vi "Retest.vi"(0 "Image In":T1, 1 "Image Dst":T1, 7 "error in":errorcluster) -> (20 "Image Out":T1, 21 "Objects (pixel) (Object Tracking 1)":T2(array[cluster]), 22 "Objects (real-world) (Object Tracking 1)":T2(array[cluster]), 27 "error out":errorcluster)   [LabVIEW 2016]
doc: "Creates, edits, and runs vision algorithms using NI Vision Assistant.\n\nWhen you place this Express VI on the block diagram, NI Vision Assistant launches. Create an algorithm using the Vision Assistant processing functions. After you create an algorithm, you can select the controls and indicators that you want to be able to programmatically set in LabVIEW. Double-click the Vision Assistant Express VI to edit the algorithm."
uses:
  <vilib>/vision/Image Controls.llb/IMAQ Image.ctl
  <vilib>/vision/Tracking.llb/IMAQ Object Tracking SessionType.ctl
  <vilib>/vision/Vision Assistant Utils.llb/IVA Object Tracking - Init Function.ctl
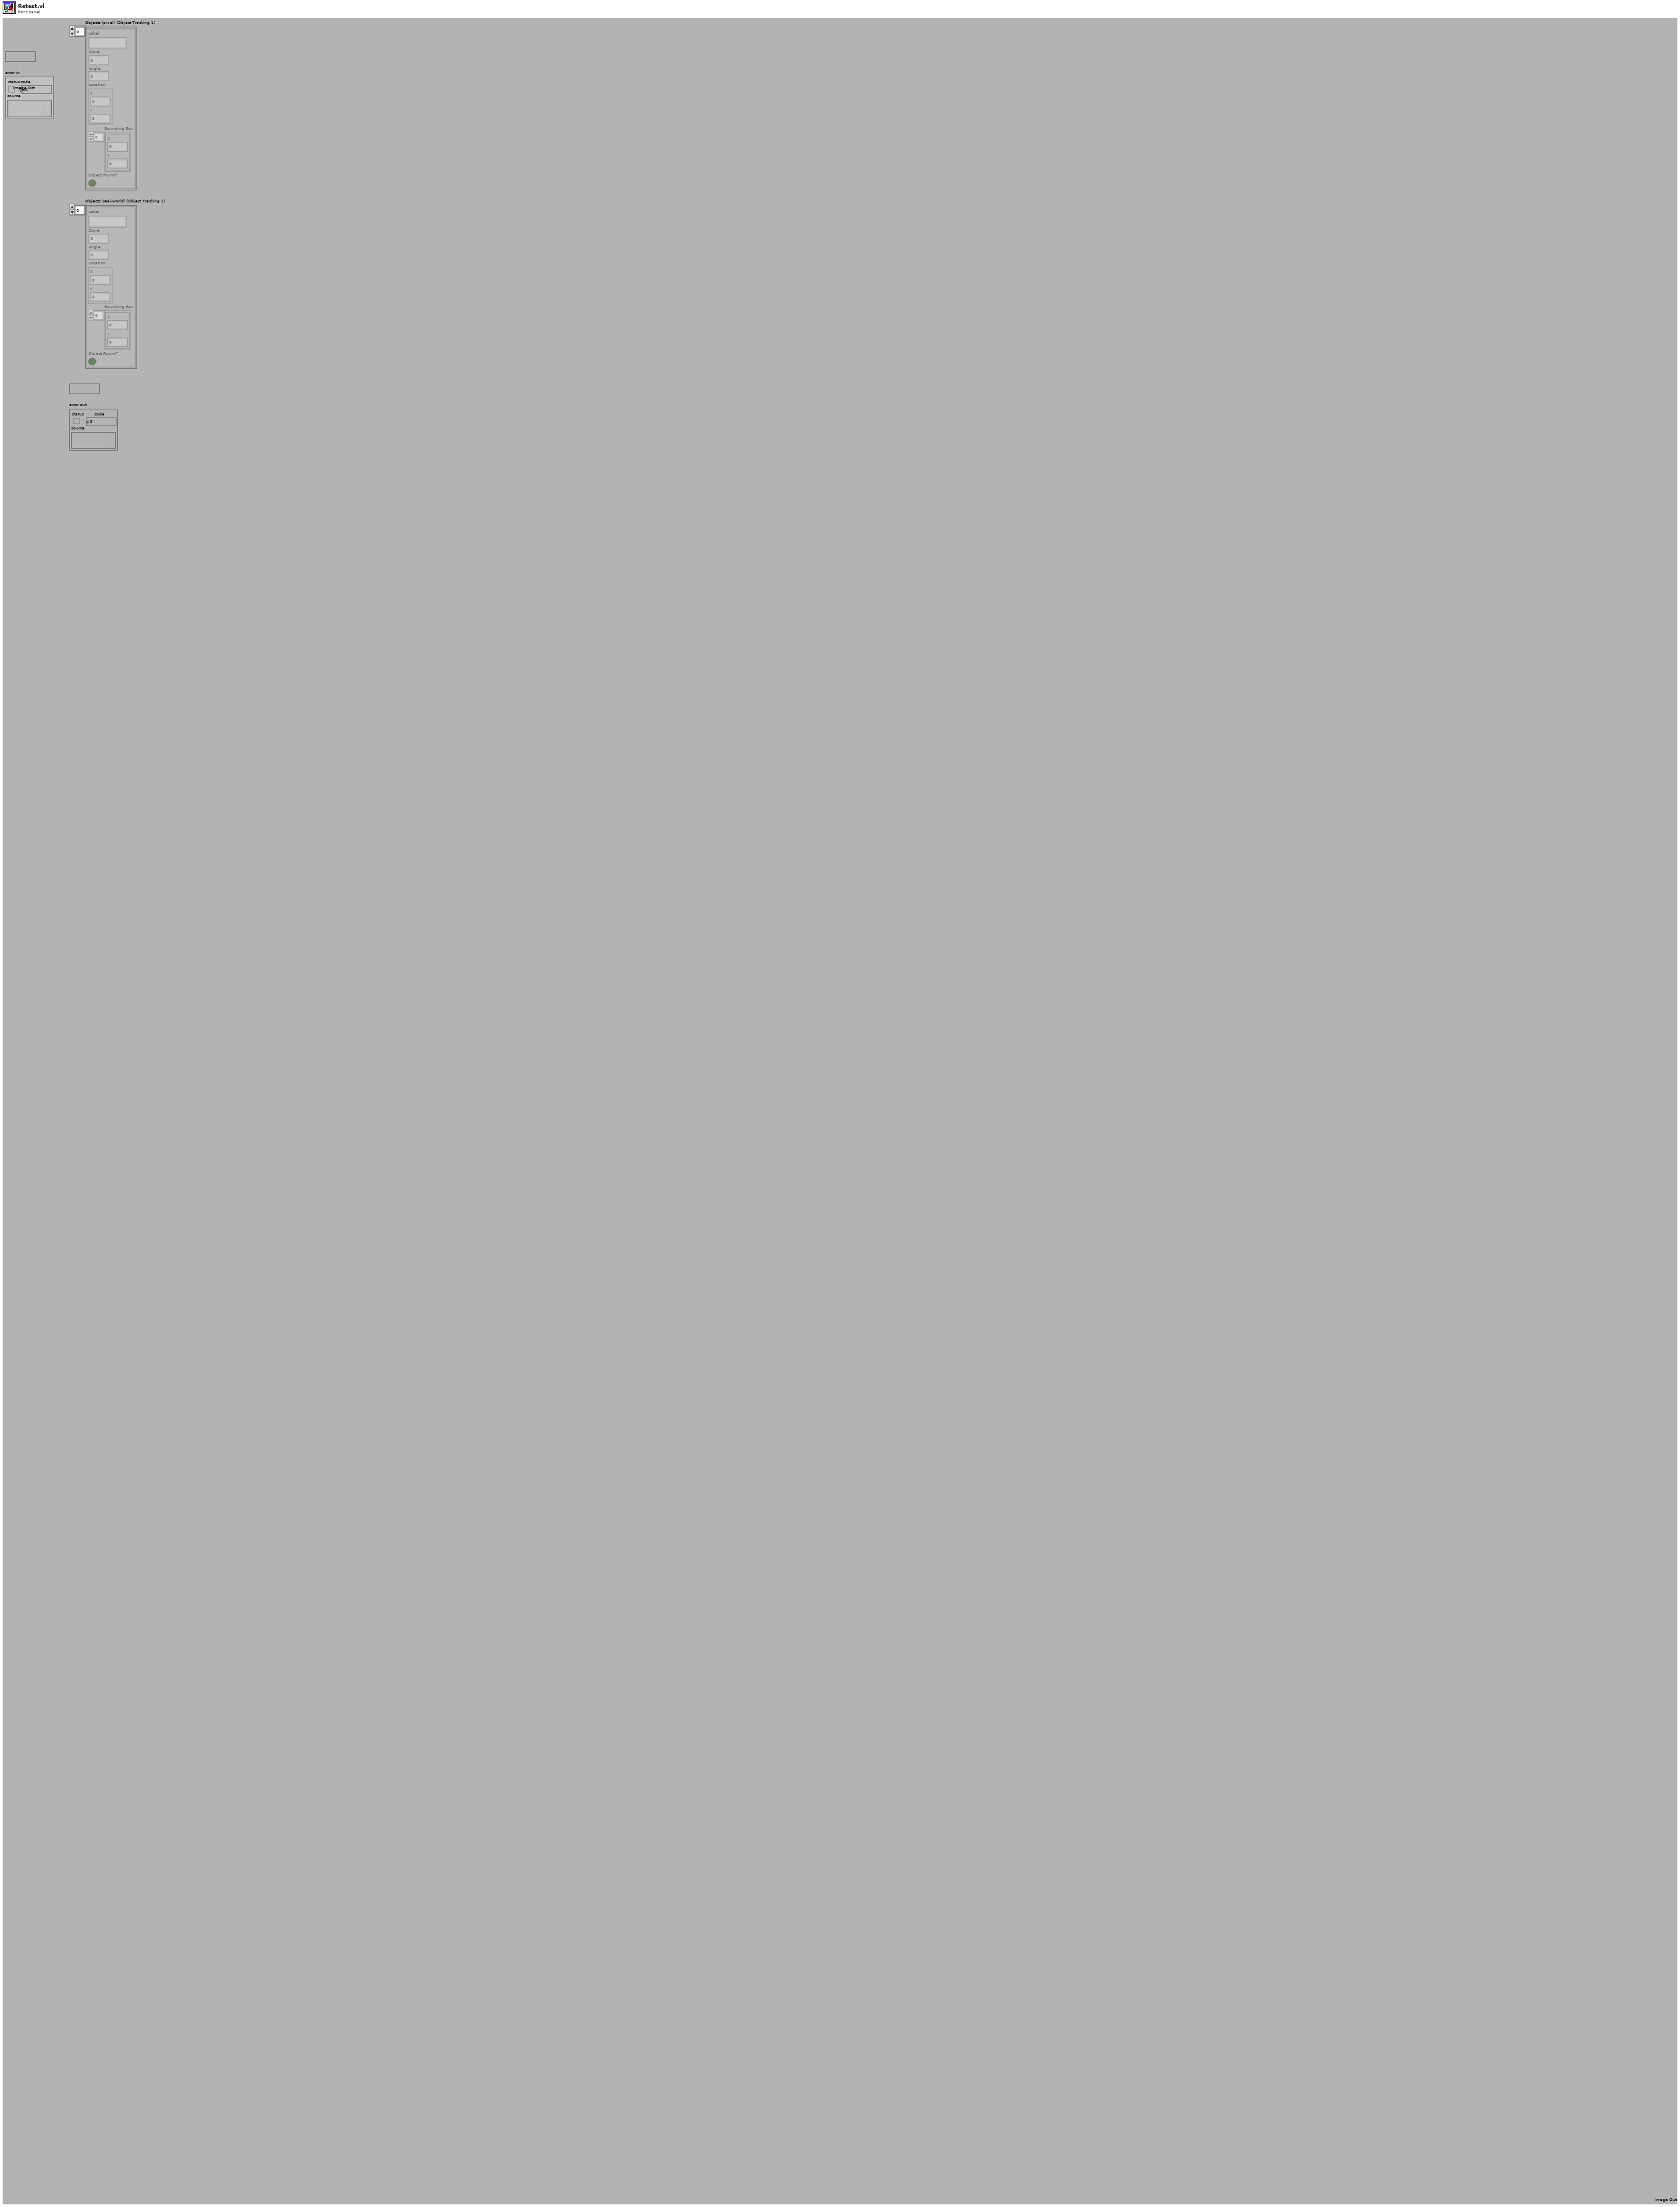
[diagram p1: front panel]
types:
  T1 = typedef "IMAQ Image.ctl" = refnum<image>
  T2 = cluster{"Label":string, "Score":i32, "Angle":dbl, "Location":cluster{"X":dbl, "Y":dbl}, "Bounding Box":cluster{"X":dbl, "Y":dbl}[], "Object Found?":bool}[]
  T3 = cluster{"Number of Histogram Bins":i32, "Blending Parameter (%)":dbl, "Max Scale Change (%)":dbl, "Max Rotation Change":dbl, "Max Shape Change (%)":dbl, "Maximum Iterations":i32}
  T4 = typedef "IVA Object Tracking - Init Function.ctl" = enum16{"Init", "Get", "Set"}
  T5 = cluster{"Initial Position":cluster{"Source":enum16{"Constant", "Measure"}, "Point ID":cluster{"GUID":string, "Index":i32}, "Point":cluster{"x":sgl, "y":sgl}}, "Initial Angle":cluster{"Source":enum16{"Constant", "Measure"}, "Measure ID":cluster{"GUID":string, "Index":i32}, "Value":dbl}}[]
  T6 = typedef "IMAQ Object Tracking SessionType.ctl" = i32
  T7 = typedef "Image Type" = u32
  T8 = cluster{"Number of Histogram Bins":i32, "Blending Parameter (%)":dbl, "Maximum Iterations":i32}
  T9 = typedef "IMAQ Object Tracking Session.ctl" = refnum<k20>
  T10 = cluster{"Source":enum16{"Constant", "Measure"}, "Point ID":cluster{"GUID":string, "Index":i32}, "Point":cluster{"x":sgl, "y":sgl}}
  T11 = cluster{"Source":enum16{"Constant", "Measure"}, "Measure ID":cluster{"GUID":string, "Index":i32}, "Value":dbl}
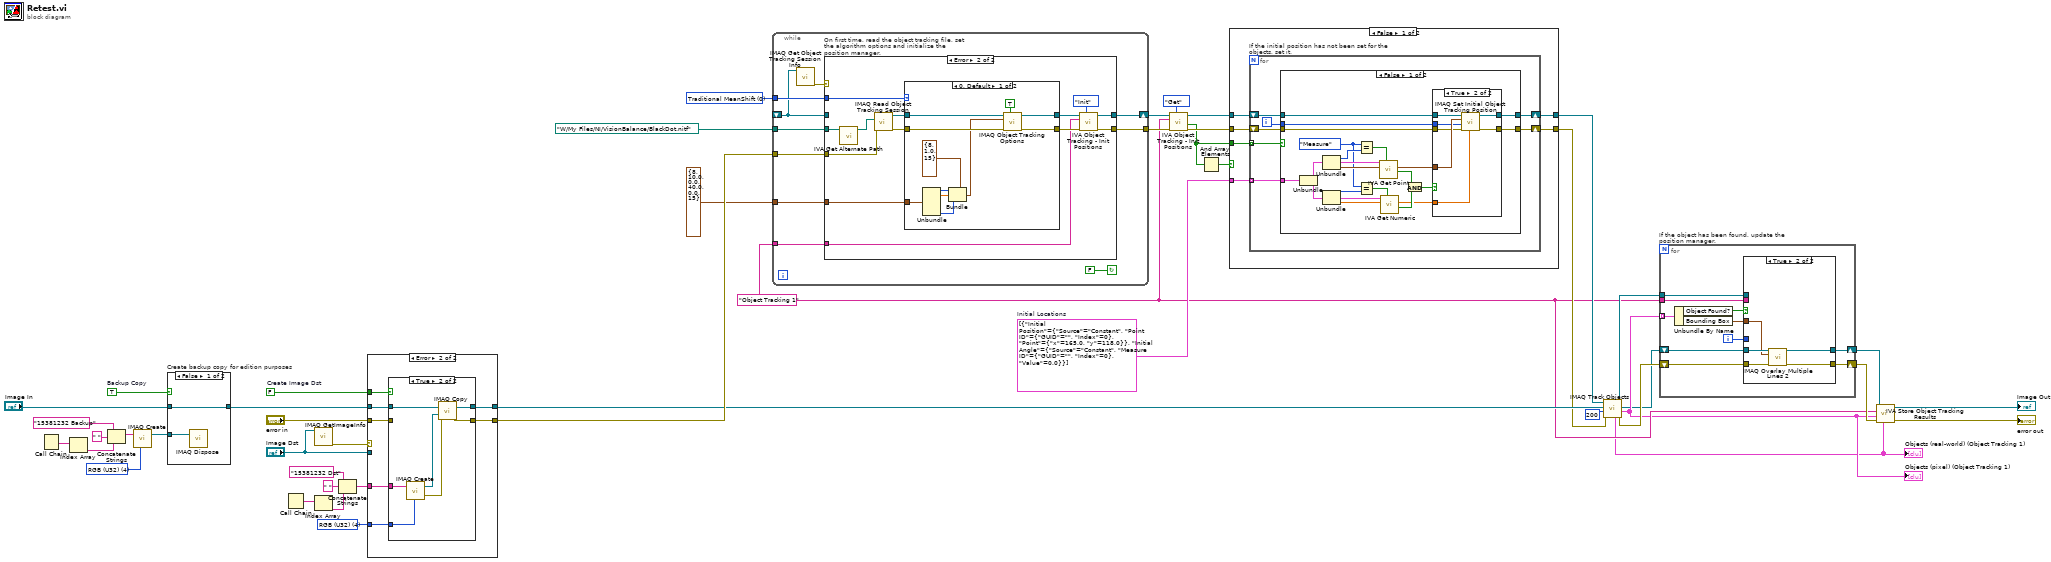
[diagram p0: block diagram]
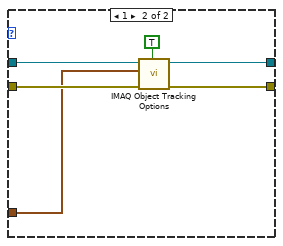
[diagram p7: hidden frame]
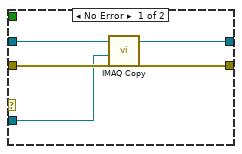
[diagram p8: hidden frame]
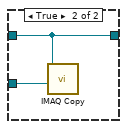
[diagram p10: hidden frame]
diagram:
  w7 = "Object Tracking 1" ("Step Name")
  w21 = T5 [{"Initial Position"={"Source"=enum."Constant", "Point ID"={"GUID"="", "Index"=0}, "Point"={"x"=165.0, "y"=118.0}}, "Initial Angle"={"Source"=enum."Constant", "Measure ID"={"GUID"="", "Index"=0}, "Value"=0.0}}]  # Initial Locations
  w23 = T6 0 items=["Traditional MeanShift", "Shape Adapted MeanShift"] ("Algorithm")
  w26 = T7 4 items=["Grayscale (U8)", "Grayscale (I16)", "Grayscale (SGL)", "Complex (CSG)", "RGB (U32)", "HSL (U32)", "RGB (U64)", "Grayscale (U16)"] ("Image Dst Type")
  w27 = T7 4 items=["Grayscale (U8)", "Grayscale (I16)", "Grayscale (SGL)", "Complex (CSG)", "RGB (U32)", "HSL (U32)", "RGB (U64)", "Grayscale (U16)"] ("Image Type")
  w46 = TRUE  # Backup Copy
  w39 = FALSE  # Create Image Dst
  n1 = Call Chain() -> (call chain=w33:string[])
  n2 = Index Array(array=w33) -> (element=w32:string)  [unwired: 1 in]
  n3 = Concatenate Strings("15381232 Backup" ("Backup Image Name"), " ", w32) -> (w29:string)
  n4 = call "IMAQ Create"("Image Name"=w29, "Image Type"=w27) -> ("New Image"=w28:T1)  [unwired: 2 in, 2 out]
  n5 = case "Create backup copy for edition purposes" shown="False" w46 {
    tunnel: [w48 w50] -> w42
    tunnel: "Image In" -> [w48 w50]
    tunnel: w28 -> [w47 w49]
    frame False {
      n6 = call "IMAQ Dispose"("Image"=w47) -> ()  [unwired: 2 in, 4 out]
    }
    frame True {
      n7 = call "IMAQ Copy"("Image Dst"=w49, "Image Src"=w50) -> ()  [unwired: 1 in, 5 out]
    }
  }
  n8 = Call Chain() -> (call chain=w38:string[])
  n9 = call "IMAQ GetImageInfo"("Image"="Image Dst") -> ("error out"=w44:errorcluster)  [unwired: 1 in, 9 out]
  n10 = Index Array(array=w38) -> (element=w36:string)  [unwired: 1 in]
  n11 = Concatenate Strings("15381232 Dst" ("Image Dst Name"), " ", w36) -> (w34:string)
  n12 = case shown="Error" w44 {
    tunnel: [w55 w59] -> w24
    tunnel: [w54 w58] -> w40
    tunnel: w42 -> [w53 w60]
    tunnel: "error in" -> [w52 w56]
    tunnel: "Image Dst" -> [w51 _]
    tunnel: w34 -> [_ w62]
    tunnel: w26 -> [_ w61]
    tunnel: w39 -> [_ w57]
    frame No Error {
      n13 = call "IMAQ Copy"("error in (no error)"=w52, "Image Dst"=w51, "Image Src"=w53) -> ("error out"=w54:errorcluster, "Image Dst Out"=w55:T1)  [unwired: 3 out]
    }
    frame Error {
      n14 = case shown="True" w57 {
        tunnel: w62 -> [_ w71]
        tunnel: w61 -> [_ w70]
        tunnel: w60 -> [w64 w68]
        tunnel: [w64 w67] -> w59
        tunnel: [w63 w66] -> w58
        tunnel: w56 -> [w63 _]
        frame False {
        }
        frame True {
          n15 = call "IMAQ Create"("Image Name"=w71, "Image Type"=w70) -> ("New Image"=w69:T1, "error out"=w65:errorcluster)  [unwired: 2 in, 1 out]
          n16 = call "IMAQ Copy"("error in (no error)"=w65, "Image Dst"=w69, "Image Src"=w68) -> ("error out"=w66:errorcluster, "Image Dst Out"=w67:T1)  [unwired: 3 out]
        }
      }
    }
  }
  n17 = while {
    shift-right: [w81] -> w19
    shift-left: _ -> [w72]
    tunnel: path "W:/My Files/NI/VisionBalance/BlackDot.nitf" ("Tracking Session File Path") -> [w79]
    tunnel: w40 -> [w78]
    tunnel: w23 -> [w77]
    tunnel: [w76] -> w16
    tunnel: T3 {"Number of Histogram Bins"=8, "Blending Parameter (%)"=10.0, "Max Scale Change (%)"=0.0, "Max Rotation Change"=40.0, "Max Shape Change (%)"=0.0, "Maximum Iterations"=15} ("Options") -> [w75]
    tunnel: w7 -> [w74]
    stop <- FALSE continue-if-true
    n18 = call "IMAQ Get Object Tracking Session Info"("Object Tracking Session In"=w72) -> ("error out"=w73:errorcluster)  [unwired: 1 in, 9 out]
    n19 = case "On first time, read the object tracking file, set the algorithm options and initialize the position manager." shown="Error" w73 {
      tunnel: [w83 w88] -> w81
      tunnel: w72 -> [w83 _]
      tunnel: w79 -> [_ w96]
      tunnel: w78 -> [w82 w94]
      tunnel: w77 -> [_ w93]
      tunnel: [w82 w87] -> w76
      tunnel: w75 -> [_ w90]
      tunnel: w74 -> [_ w84]
      frame No Error {
      }
      frame Error {
        n20 = call <vilib>:"IVA Get Alternate Path.vi"("Path In"=w96) -> ("Path Out"=w95:path)  [unwired: 10 out]
        n21 = call "IMAQ Read Object Tracking Session"("error in (no error)"=w94, "Object Tracking Session File Path"=w95) -> ("error out"=w91:errorcluster, "Object Tracking Session Out"=w92:T9)  [unwired: 1 in, 7 out]
        n22 = case shown="0, Default" w93 {
          tunnel: w92 -> [w107 w113]
          tunnel: [w106 w112] -> w89
          tunnel: w91 -> [w105 w111]
          tunnel: [w104 w110] -> w86
          tunnel: w90 -> [w103 w109]
          frame 0, Default {
            n23 = Unbundle(w103) -> ("Number of Histogram Bins"=w102:i32, "Blending Parameter (%)"=w101:dbl, "Maximum Iterations"=w97:i32)  [unwired: 3 out]
            n24 = Bundle(cluster=T8 {"Number of Histogram Bins"=8, "Blending Parameter (%)"=1.0, "Maximum Iterations"=15} ("Mean Shift Options in"), "Number of Histogram Bins"=w102, "Blending Parameter (%)"=w101, "Maximum Iterations"=w97) -> (w100:T8)
            n25 = call-poly "IMAQ Object Tracking Options"("Get/Set (Get)"=TRUE, "error in (no error)"=w105, "Mean Shift Options in"=w100, "Object Tracking Session In"=w107) -> ("error out"=w104:errorcluster, "Object Tracking Session Out"=w106:T9)  [unwired: 1 in, 5 out]
          }
          frame 1 {
            n26 = call-poly "IMAQ Object Tracking Options"("Get/Set (Get)"=TRUE, "error in (no error)"=w111, "Shape Adapted Options in"=w109, "Object Tracking Session In"=w113) -> ("error out"=w110:errorcluster, "Object Tracking Session Out"=w112:T9)  [unwired: 2 in, 4 out]
          }
        }
        n27 = call <vilib>:"IVA Object Tracking - Init Positions.vi"("Function"=IVA_Object_Tracking_-_Init_Function."Init", "error in (no error)"=w86, "Process ID"=w84, "Object Tracking Session In"=w89) -> ("error out"=w87:errorcluster, "Object Tracking Session dup"=w88:T9)  [unwired: 2 in, 4 out]
      }
    }
  }
  n28 = call <vilib>:"IVA Object Tracking - Init Positions.vi"("Function"=IVA_Object_Tracking_-_Init_Function."Get", "error in (no error)"=w16, "Process ID"=w7, "Object Tracking Session In"=w19) -> ("error out"=w15:errorcluster, "Init Values Out"=w13:bool[], "Object Tracking Session dup"=w18:T9)  [unwired: 2 in, 3 out]
  n29 = And Array Elements(Boolean array=w13) -> (logical AND=w14:bool)
  n30 = case shown="False" w14 {
    tunnel: w21 -> [w119 _]
    tunnel: [w118 w161] -> w20
    tunnel: w18 -> [w117 w161]
    tunnel: w15 -> [w116 w160]
    tunnel: w13 -> [w115 _]
    tunnel: [w114 w160] -> w12
    frame False {
      n31 = for "If the initial position has not been set for the objects, set it." {
        tunnel: w119 -> [w125] mode=indexing
        shift-right: [w123] -> w118
        shift-left: w117 -> [w126]
        shift-right: [w120] -> w114
        shift-left: w116 -> [w122]
        tunnel: w115 -> [w121] mode=indexing
        i -> [w124]
        n32 = case shown="False" w121 {
          tunnel: w126 -> [w148 w159]
          tunnel: w125 -> [w147 _]
          tunnel: w124 -> [w131 _]
          tunnel: [w129 w159] -> w123
          tunnel: w122 -> [w128 w158]
          tunnel: [w127 w158] -> w120
          frame False {
            w137 = enum16{"Constant", "Measure"}."Measure" ("Source")
            n33 = Unbundle(w147) -> ("Initial Position"=w146:T10, "Initial Angle"=w145:T11)
            n34 = Unbundle(w146) -> ("Source"=w140:enum16{"Constant", "Measure"}, "Point ID"=w144:cluster{"GUID":string, "Index":i32}, "Point"=w143:cluster{"x":sgl, "y":sgl})
            n35 = Unbundle(w145) -> ("Source"=w138:enum16{"Constant", "Measure"}, "Measure ID"=w142:cluster{"GUID":string, "Index":i32}, "Value"=w141:dbl)
            n36 = Equal?(x=w137, y=w140) -> (x = y?=w139:bool)
            n37 = Equal?(x=w137, y=w138) -> (x = y?=w136:bool)
            n38 = call <vilib>:"IVA Get Point.vi"("Point Source"=w139, "Point in"=w143, "Point ID"=w144) -> ("Available?"=w135:bool, "Point out"=w132:cluster{"x":sgl, "y":sgl})  [unwired: 1 in, 6 out]
            n39 = call <vilib>:"IVA Get Numeric.vi"("Source"=w136, "Numeric in"=w141, "Result ID"=w142) -> ("Available?"=w134:bool, "Numeric out"=w130:dbl)  [unwired: 1 in, 6 out]
            n40 = And(x=w135, y=w134) -> (x .and. y?=w133:bool)
            n41 = case shown="True" w133 {
              tunnel: w148 -> [w150 w157]
              tunnel: w132 -> [_ w156]
              tunnel: w131 -> [_ w155]
              tunnel: w130 -> [_ w151]
              tunnel: [w150 w154] -> w129
              tunnel: w128 -> [w149 w153]
              tunnel: [w149 w152] -> w127
              frame False {
              }
              frame True {
                n42 = call "IMAQ Set Initial Object Tracking Position"("Initial Angle"=w151, "error in (no error)"=w153, "Object Index"=w155, "Position"=w156, "Object Tracking Session In"=w157) -> ("error out"=w152:errorcluster, "Object Tracking Session Out"=w154:T9)  [unwired: 5 out]
              }
            }
          }
          frame True {
          }
        }
      }
    }
    frame True {
    }
  }
  n43 = call "IMAQ Track Objects"("error in (no error)"=w12, "Minimum Score"=200, "Image"=w24, "Object Tracking Session In"=w20) -> ("error out"=w11:errorcluster, "Objects (pixel)"=w6:T2, "Image (duplicate)"=w3:T1, "Object Tracking Session Out"=w10:T9, "Objects (real-world)"=w5:T2)  [unwired: 3 out]
  "Objects (pixel) (Object Tracking 1)" <- w6
  "Objects (real-world) (Object Tracking 1)" <- w5
  n44 = for "If the object has been found, update the position manager." {
    tunnel: w6 -> [w171] mode=indexing
    tunnel: w7 -> [w170]
    shift-right: [w167] -> w9
    shift-left: w11 -> [w164]
    tunnel: w10 -> [w169]
    shift-right: [w163] -> w2
    shift-left: w3 -> [w165]
    i -> [w166]
    n45 = Unbundle By Name(w171) -> ("Object Found?"=w168:bool, "Bounding Box"=w162:cluster{"X":dbl, "Y":dbl}[])
    n46 = case shown="True" w168 {
      tunnel: w170 -> [_ _]
      tunnel: w169 -> [_ _]
      tunnel: [w173 w177] -> w167
      tunnel: w166 -> [_ _]
      tunnel: w165 -> [w172 w178]
      tunnel: w164 -> [w173 w176]
      tunnel: [w172 w175] -> w163
      tunnel: w162 -> [_ w174]
      frame False {
      }
      frame True {
        n47 = call "IMAQ Overlay Multiple Lines 2"("Image"=w178, "Line End Points"=w174, "error in (no error)"=w176) -> ("Image Out"=w175:T1, "error out"=w177:errorcluster)  [unwired: 11 in]
      }
    }
  }
  n48 = call <vilib>:"IVA Store Object Tracking Results.vi"("Objects (real-world)"=w5, "error in (no error)"=w9, "Objects (pixel)"=w6, "Step Name"=w7, "Image in"=w2) -> ("error out"=→"error out":errorcluster, "Image dup"=→"Image Out":T1)  [unwired: 5 out]
